vi "Averaged FFT Spectrum (Mag-Phase).vi"(0 "scaled signal [EU]":dbl[](array[numeric]) format="%.2f", 1 "sampling frequency [Hz]":dbl=10000.0 format="%.2f", 2 "window":T7 items=["Rectangle"=0, "Hanning"=1, "Hamming"=2, "Blackman-Harris"=3, "Exact Blackman"=4, "Blackman"=5, "Flat Top"=6, "4 Term B-Harris "=7, "7 Term B-Harris"=8, "Low Sidelobe"=9, "Blackman Nuttall"=11, "Triangle"=30, "Bartlett-Hanning"=31, "Bohman"=32, "Parzen"=33, "Welch"=34, "Kaiser"=60, "Dolph-Chebyshev"=61, "Gaussian"=62], 4 "view":T4, 5 "channel info":T1={"sensor sensitivity [mV/EU]"=1000.0, "engineering units"=1, "dB reference [EU]"=1.0, "custom label"="EU", "weighting filter"=0, "pregain [dB]"=0.0} {"pregain [dB]" format="%.2f"; "weighting filter" items=["Linear", "A-weighting", "B-weighting", "C-weighting", "ITU-R 468-4", "Dolby", "CCITT", "C-message"]; "dB reference [EU]" format="%^.1e"; "engineering units" items=["custom..."=0, "V"=1, "A"=21, "Pa"=2, "N"=20, "g"=3, "m/s^2"=4, "m/s"=5, "m"=6, "mm/s"=12, "mm"=13, "microns/s"=14, "microns"=15, "in/s^2"=7, "in/s"=8, "in"=9, "mils/s"=10, "mils"=11, "rad/s^2"=16, "rad/s"=17, "rad"=18, "strain"=19]; "sensor sensitivity [mV/EU]" format="%.2f"}, 6 "frequency weighting":T6(ring), 7 "reset averaging (T)":bool=TRUE, 9 "averaging parameters":T5={"averaging mode"=enum."RMS averaging", "weighting mode"=enum."Linear", "number of averages"=10} {"number of averages" min=1}) -> (11 "window constants":cluster{"eq noise BW":dbl, "coherent gain":dbl} {"coherent gain" format="%.2f"; "eq noise BW" format="%.2f"}, 12 "df [Hz]":dbl format="%.2f", 13 "weighting conflict":bool, 14 "magnitude [EUrms]":dbl[](array[numeric]) format="%.2f", 15 "unit label (magnitude)":string, 16 "phase":dbl[](array[numeric]) format="%.2f", 17 "unit label (phase)":string, 18 "averages completed":dbl format="%.2f", 19 "error out":errorcluster)   [LabVIEW 2017]
doc: "Computes the averaged FFT spectrum of the input signal. FFT results are returned as magnitude and phase.\nEach block of data corresponds to a single FFT block and has to be passed individually to this VI. The first time this VI is called, reset averaging must be TRUE (default value), to start a new averaging process. For subsequent calls, reset averaging must be FALSE to continue the averaging process. Averages completed returns the number of averages completed so far.\nAveraging parameters specifies how the averaging is performed. This includes the averaging mode (no averaging, vector averaging, RMS averaging, or peak hold), the weighting mode (linear or exponential), and the number of averages (used only if the weighting mode is exponential).\nThe view cluster allows you to display magnitude results in decibels, and the phase results unwrapped or not, in radians or degrees.\nThe selected frequency weighting (A, B, or C) is applied to the results in the frequency domain. There is no time-domain filtering operation."
uses:
  <vilib>/Analysis/4window.llb/windowTd.ctl
  <vilib>/addons/Sound and Vibration/compatibility/Controls/svl_Channel Info.ctl
  <vilib>/addons/Sound and Vibration/compatibility/Controls/svl_Engineering Units Text Ring.ctl
  <vilib>/addons/Sound and Vibration/compatibility/Controls/svl_Weighting Filter Text Ring.ctl
  <vilib>/Analysis/2dsp.llb/Real FFT.vi
  <vilib>/Analysis/2dsp.llb/Power Spectrum (DBL).vi
  <vilib>/Analysis/0measdsp.llb/Scaled Time Domain Window (DBL).vi
  <vilib>/Analysis/NI_AALPro.lvlib
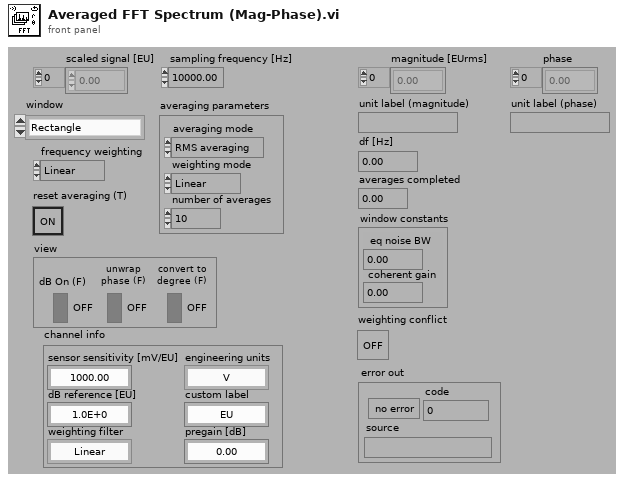
[diagram p1: front panel]
types:
  T1 = typedef "svl_Channel Info.ctl" = cluster{"sensor sensitivity [mV/EU]":dbl, "engineering units":T2, "dB reference [EU]":dbl, "custom label":string, "weighting filter":T3, "pregain [dB]":dbl}
  T2 = typedef "svl_Engineering Units Text Ring.ctl" = u16
  T3 = typedef "svl_Weighting Filter Text Ring.ctl" = u16
  T4 = cluster{"dB On (F)":bool, "unwrap phase (F)":bool, "convert to degree (F)":bool}
  T5 = cluster{"averaging mode":enum16{"No averaging", "Vector averaging", "RMS averaging", "Peak hold"}, "weighting mode":enum16{"Linear", "Exponential"}, "number of averages":u32}
  T6 = enum16{"Linear", "A-weighting", "B-weighting", "C-weighting"}
  T7 = typedef "NI_AALPro.lvlib/windowTd.ctl" = u32
  T8 = enum16{"No averaging", "Vector averaging", "RMS averaging", "Peak hold"}
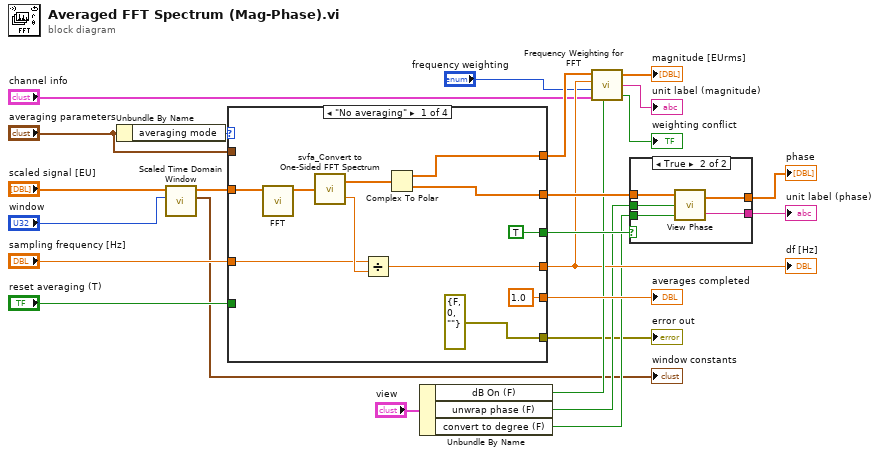
[diagram p0: block diagram]
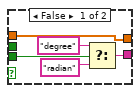
[diagram p2: hidden frame]
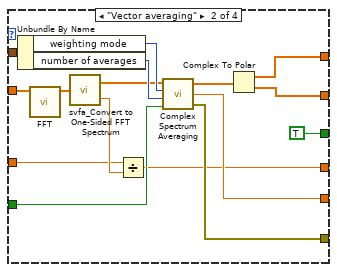
[diagram p3: hidden frame]
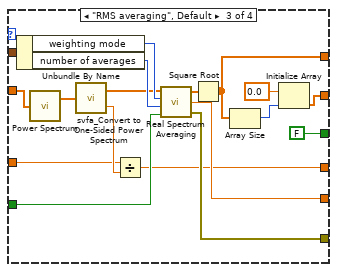
[diagram p4: hidden frame]
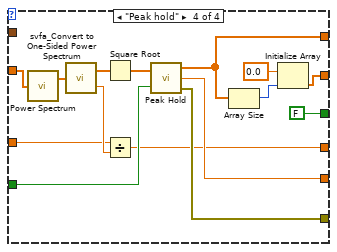
[diagram p5: hidden frame]
diagram:
  n1 = Unbundle By Name("averaging parameters") -> ("averaging mode"=w20:T8)
  n2 = call-poly <vilib>:"Scaled Time Domain Window.vi"("window"="window", "X"="scaled signal [EU]") -> ("window properties"=→"window constants":cluster{"eq noise BW":dbl, "coherent gain":dbl}, "Windowed X"=w21:dbl[])  [unwired: 7 in, 1 out]
  n3 = case shown="\"No averaging\"" w20 {
    tunnel: "sampling frequency [Hz]" -> [w27 w38 w54 w73]
    tunnel: [w26 w37 w53 w72] -> w11
    tunnel: [1.0 ("averages completed") w52 w69 w83] -> w24
    tunnel: "reset averaging (T)" -> [_ w51 w70 w84]
    tunnel: w21 -> [w29 w40 w56 w74]
    tunnel: "averaging parameters" -> [_ w50 w68 _]
    tunnel: [w35 w48 w60 w79] -> w17
    tunnel: [w34 w47 w67 w80] -> w18
    tunnel: [TRUE TRUE FALSE FALSE] -> w16
    tunnel: [errorcluster {"status"=FALSE, "code"=0, "source"=""} ("error out") w43 w63 w77] -> w3
    frame "No averaging" {
      n4 = call-poly <vilib>:"FFT.vi"("X"=w29) -> ("FFT {X}"=w31:cdb[])  [unwired: 9 in, 1 out]
      n5 = call <vilib>:"svfa_Convert to One-Sided FFT Spectrum.vi"("two-sided FFT spectrum"=w31) -> ("one-sided FFT spectrum"=w28:cdb[], "block size"=w30:dbl)
      n6 = Divide(x=w27, y=w30) -> (x/y=w26:dbl)
      n7 = Complex To Polar(r * e^(i*theta)=w28) -> (r=w35:dbl[], theta=w34:dbl[])
    }
    frame "Vector averaging" {
      n8 = Unbundle By Name(w50) -> ("weighting mode"=w45:enum16{"Linear", "Exponential"}, "number of averages"=w44:u32)
      n9 = call-poly <vilib>:"FFT.vi"("X"=w40) -> ("FFT {X}"=w42:cdb[])  [unwired: 9 in, 1 out]
      n10 = call <vilib>:"svfa_Convert to One-Sided FFT Spectrum.vi"("two-sided FFT spectrum"=w42) -> ("one-sided FFT spectrum"=w39:cdb[], "block size"=w41:dbl)
      n11 = Divide(x=w38, y=w41) -> (x/y=w37:dbl)
      n12 = call <vilib>:"Complex Spectrum Averaging.vi"("reset averaging (T)"=w51, "number of averages"=w44, "weighting mode"=w45, "complex spectrum"=w39) -> ("error out"=w43:errorcluster, "averages completed"=w52:dbl, "averaged complex spectrum"=w49:cdb[])
      n13 = Complex To Polar(r * e^(i*theta)=w49) -> (r=w48:dbl[], theta=w47:dbl[])
    }
    frame "RMS averaging", Default {
      n14 = Unbundle By Name(w68) -> ("weighting mode"=w59:enum16{"Linear", "Exponential"}, "number of averages"=w62:u32)
      n15 = call-poly <vilib>:"Power Spectrum.vi"("X"=w56) -> ("Power Spectrum"=w58:dbl[])  [unwired: 1 out]
      n16 = call <vilib>:"svfa_Convert to One-Sided Power Spectrum.vi"("two-sided power spectrum"=w58) -> ("one-sided power spectrum"=w55:dbl[], "block size"=w57:dbl)
      n17 = Divide(x=w54, y=w57) -> (x/y=w53:dbl)
      n18 = call <vilib>:"Real Spectrum Averaging.vi"("reset averaging (T)"=w70, "number of averages"=w62, "weighting mode"=w59, "real spectrum"=w55) -> ("error out"=w63:errorcluster, "averages completed"=w69:dbl, "averaged real spectrum"=w61:dbl[])
      n19 = Square Root(x=w61) -> (sqrt(x)=w60:dbl[])
      n20 = Array Size(array=w60) -> (size(s)=w65:i32)
      n21 = Initialize Array(0.0, w65) -> (w67:dbl[])
    }
    frame "Peak hold" {
      n22 = call-poly <vilib>:"Power Spectrum.vi"("X"=w74) -> ("Power Spectrum"=w76:dbl[])  [unwired: 1 out]
      n23 = call <vilib>:"svfa_Convert to One-Sided Power Spectrum.vi"("two-sided power spectrum"=w76) -> ("one-sided power spectrum"=w71:dbl[], "block size"=w75:dbl)
      n24 = Square Root(x=w71) -> (sqrt(x)=w85:dbl[])
      n25 = Divide(x=w73, y=w75) -> (x/y=w72:dbl)
      n26 = call <vilib>:"Peak Hold.vi"("real spectrum"=w85, "reset averaging"=w84) -> ("peak spectrum"=w79:dbl[], "averages completed"=w83:dbl, "error out"=w77:errorcluster)
      n27 = Array Size(array=w79) -> (size(s)=w81:i32)
      n28 = Initialize Array(0.0, w81) -> (w80:dbl[])
    }
  }
  "df [Hz]" <- w11
  "averages completed" <- w24
  "error out" <- w3
  n29 = Unbundle By Name("view") -> ("dB On (F)"=w14:bool, "unwrap phase (F)"=w8:bool, "convert to degree (F)"=w7:bool)
  n30 = call <vilib>:"Frequency Weighting for FFT.vi"("FFT [EUrms]"=w17, "df [Hz]"=w11, "frequency weighting"="frequency weighting", "channel info"="channel info", "dB On (F)"=w14) -> ("frequency weighted FFT [EUrms]"=→"magnitude [EUrms]":dbl[], "unit label"=→"unit label (magnitude)":string, "weighting conflict"=→"weighting conflict":bool)
  n31 = case shown="True" w16 {
    tunnel: [w90 w94] -> w10
    tunnel: w18 -> [w90 w95]
    tunnel: [w89 w93] -> w9
    tunnel: w8 -> [_ w92]
    tunnel: w7 -> [w88 w91]
    frame False {
      n32 = Select(t="degree", s=w88, f="radian") -> (s? t:f=w89:string)
    }
    frame True {
      n33 = call <vilib>:"View Phase.vi"("convert to degree (F)"=w91, "unwrap phase (F)"=w92, "phase (radian)"=w95) -> ("unit label (phase)"=w93:string, "scaled phase"=w94:dbl[])
    }
  }
  "phase" <- w10
  "unit label (phase)" <- w9
